vi "Link VChannel.vi"(4 "Channel State":cluster{bool, bool, bool, bool}, 5 "error in (no error)":errorcluster, 7 "VISA resource name":refnum<visa-resource-name>="DSOS404") -> (1 "error out":errorcluster, 2 "Waveform Graph":waveform(dbl)[](graph), 3 "VISA resource name out":refnum<visa-resource-name>)   [LabVIEW 2018]
uses:
  <instrlib>/Agilent 90000 Series/Agilent 90000 Series.lvlib
panel:
  # "CH1"
  # "CH2"
  # "CH3"
  # "CH4"
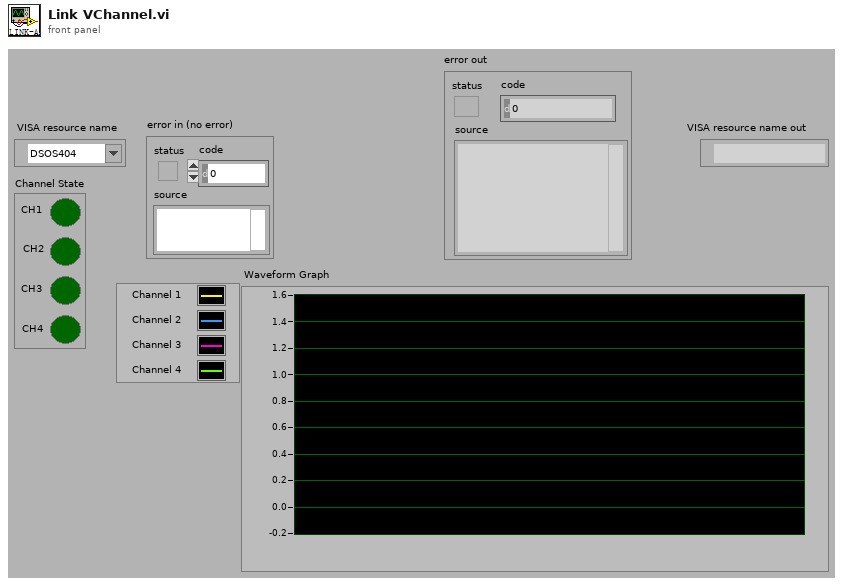
[diagram p1: front panel]
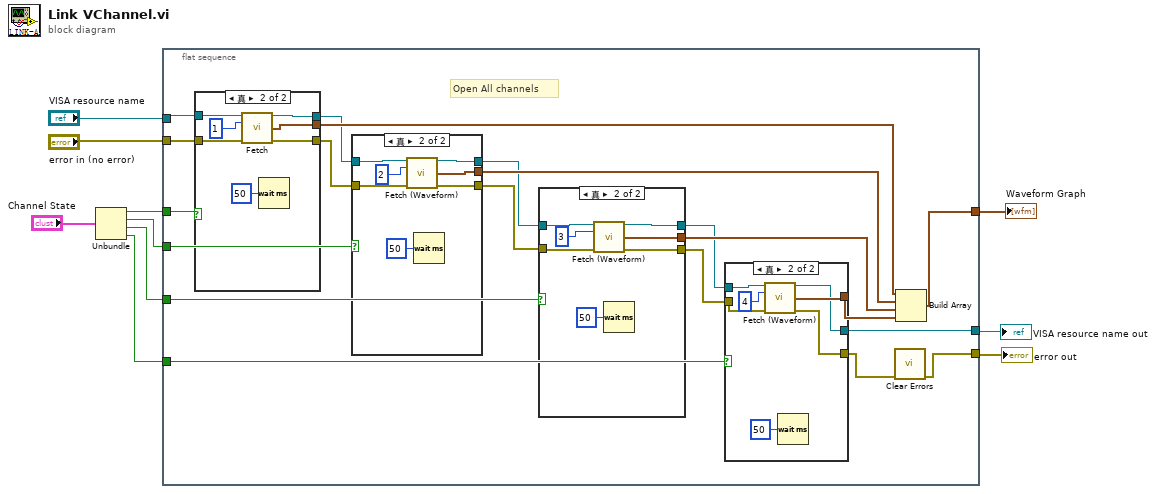
[diagram p0: block diagram]
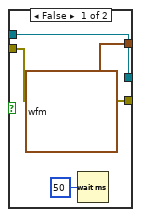
[diagram p2: hidden frame]
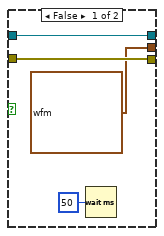
[diagram p3: hidden frame]
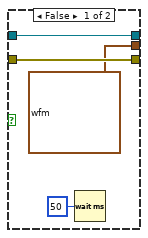
[diagram p4: hidden frame]
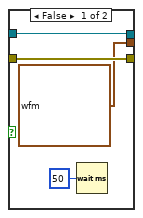
[diagram p5: hidden frame]
diagram:
  n1 = Unbundle("Channel State") -> (w7:bool, w6:bool, w5:bool, w4:bool)
  n2 = flat-sequence {
    tunnel: [w26] -> w10
    tunnel: [w11] -> w9
    tunnel: [w25] -> w8
    tunnel: "VISA resource name" -> [w18]
    tunnel: "error in (no error)" -> [w17]
    tunnel: w7 -> [w16]
    tunnel: w6 -> [w15]
    tunnel: w5 -> [w14]
    tunnel: w4 -> [w13]
    frame #0 {
      # "Open All channels"
      n3 = case shown="真" w16 {
        tunnel: w18 -> [w67 w74]
        tunnel: w17 -> [w66 w73]
        tunnel: [waveform(dbl) {"t0"=timestamp(0 s since 1904-01-01), "dt"=1.0, "Y"=[]} ("element") w68] -> w30
        tunnel: [w67 w72] -> w24
        tunnel: [w66 w71] -> w22
        frame False {
          n4 = Wait (ms)(milliseconds to wait=u32 50) -> ()  [unwired: 1 out]
        }
        frame True {
          n5 = call-poly <instrlib>:"Fetch.vi"("VISA resource name"=w74, "Measurement Source (1: Channel 1)"=1 ("y"), "error in (no error)"=w73) -> ("VISA resource name out"=w72:refnum<visa-resource-name>, "Waveform Data"=w68:waveform(dbl), "error out"=w71:errorcluster)  [unwired: 10 in]
          n6 = Wait (ms)(milliseconds to wait=u32 50) -> ()  [unwired: 1 out]
        }
      }
      n7 = case shown="真" w15 {
        tunnel: [waveform(dbl) {"t0"=timestamp(0 s since 1904-01-01), "dt"=1.0, "Y"=[]} ("element") w63] -> w29
        tunnel: w24 -> [w56 w62]
        tunnel: [w56 w61] -> w23
        tunnel: w22 -> [w55 w60]
        tunnel: [w55 w59] -> w21
        frame False {
          n8 = Wait (ms)(milliseconds to wait=u32 50) -> ()  [unwired: 1 out]
        }
        frame True {
          n9 = call <instrlib>:"Fetch (Waveform).vi"("VISA resource name"=w62, "Measurement Source (1: Channel 1)"=2 ("y"), "error in (no error)"=w60) -> ("VISA resource name out"=w61:refnum<visa-resource-name>, "Waveform Data"=w63:waveform(dbl), "error out"=w59:errorcluster)  [unwired: 10 in]
          n10 = Wait (ms)(milliseconds to wait=u32 50) -> ()  [unwired: 1 out]
        }
      }
      n11 = case shown="真" w14 {
        tunnel: [waveform(dbl) {"t0"=timestamp(0 s since 1904-01-01), "dt"=1.0, "Y"=[]} ("element") w52] -> w28
        tunnel: w23 -> [w45 w51]
        tunnel: [w45 w50] -> w19
        tunnel: w21 -> [w44 w49]
        tunnel: [w44 w48] -> w20
        frame False {
          n12 = Wait (ms)(milliseconds to wait=u32 50) -> ()  [unwired: 1 out]
        }
        frame True {
          n13 = call <instrlib>:"Fetch (Waveform).vi"("VISA resource name"=w51, "Measurement Source (1: Channel 1)"=3 ("y"), "error in (no error)"=w49) -> ("VISA resource name out"=w50:refnum<visa-resource-name>, "Waveform Data"=w52:waveform(dbl), "error out"=w48:errorcluster)  [unwired: 10 in]
          n14 = Wait (ms)(milliseconds to wait=u32 50) -> ()  [unwired: 1 out]
        }
      }
      n15 = case shown="真" w13 {
        tunnel: [waveform(dbl) {"t0"=timestamp(0 s since 1904-01-01), "dt"=1.0, "Y"=[]} ("element") w41] -> w27
        tunnel: [w33 w40] -> w25
        tunnel: [w32 w39] -> w12
        tunnel: w19 -> [w33 w38]
        tunnel: w20 -> [w32 w37]
        frame False {
          n16 = Wait (ms)(milliseconds to wait=u32 50) -> ()  [unwired: 1 out]
        }
        frame True {
          n17 = call <instrlib>:"Fetch (Waveform).vi"("VISA resource name"=w38, "Measurement Source (1: Channel 1)"=4 ("y"), "error in (no error)"=w37) -> ("VISA resource name out"=w40:refnum<visa-resource-name>, "Waveform Data"=w41:waveform(dbl), "error out"=w39:errorcluster)  [unwired: 10 in]
          n18 = Wait (ms)(milliseconds to wait=u32 50) -> ()  [unwired: 1 out]
        }
      }
      n19 = call <vilib>:"Clear Errors.vi"("error in (no error)"=w12) -> ("error out"=w11:errorcluster)  [unwired: 5 in, 1 out]
      n20 = Build Array(w30, w29, w28, w27) -> (w26:waveform(dbl)[])
    }
  }
  "Waveform Graph" <- w10
  "error out" <- w9
  "VISA resource name out" <- w8
